vi "CH1603_OFF All Relay.vi"(5 "Loop Read(3)":i32=3, 7 "Device Addr(0x01)":u8=1 format="%02x", 8 "error in (no error)":errorcluster, 9 "Delay Time(200ms)":u32=200, 11 "MyIndex":u8) -> (0 "error out":errorcluster, 2 "Result(T:Pass)":bool, 3 "VISA resource name out":refnum<visa-resource-name>)   [LabVIEW 2015]
doc: "Close the device all IO port(1~16 or 17~32),will set the second device IO(device address add 1);"
panel:
  out "Read String":string
  # "OFF All IO Port"
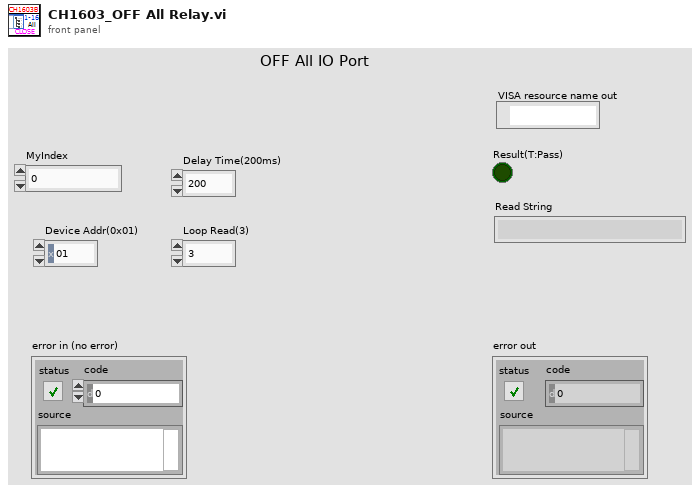
[diagram p1: front panel]
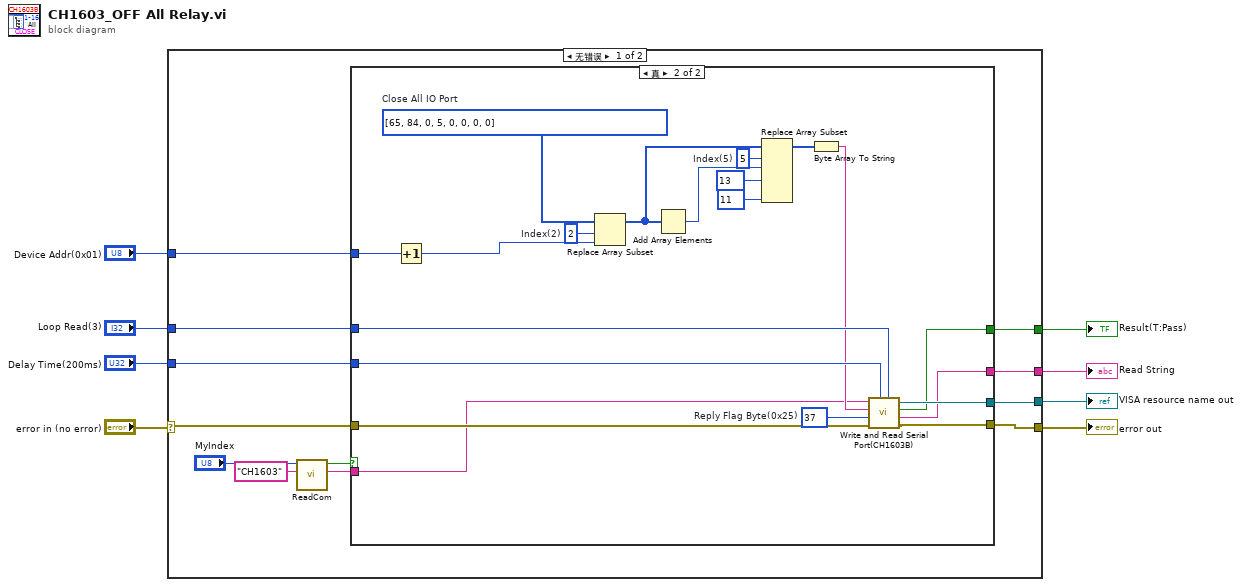
[diagram p0: block diagram]
diagram:
  n1 = case shown="无错误" "error in (no error)" {
    selector: "error in (no error)" -> [w19 w41]
    tunnel: [w18 w41] -> w6
    tunnel: [w17 _] -> w7
    tunnel: "Device Addr(0x01)" -> [w20 _]
    tunnel: "Delay Time(200ms)" -> [w16 _]
    tunnel: "Loop Read(3)" -> [w15 _]
    tunnel: [w14 _] -> w2
    tunnel: [w13 _] -> w1
    frame No Error {
      n2 = call "ReadCom.vi"("仪器名称"="CH1603", "MyIndex"="MyIndex") -> ("COM"=w9:string, "OK?"=w10:bool)  [unwired: 7 in, 1 out]
      n3 = case shown="真" w10 {
        tunnel: w20 -> [_ w34]
        tunnel: w19 -> [_ w33]
        tunnel: [_ w32] -> w18
        tunnel: [_ w31] -> w17
        tunnel: w16 -> [_ w30]
        tunnel: w15 -> [_ w29]
        tunnel: [_ w24] -> w14
        tunnel: [_ w23] -> w13
        tunnel: w9 -> [_ w21]
        frame False {
        }
        frame True {
          w25 = u8 37  # Reply Flag Byte(0x25)
          w38 = 5  # Index(5)
          w39 = 2  # Index(2)
          w40 = u8[] [65, 84, 0, 5, 0, 0, 0, 0]  # Close All IO Port
          n4 = Increment(x=w34) -> (x+1=w22:u8)
          n5 = Replace Array Subset(array=w40, new element=w22, index=w39) -> (w28:u8[])
          n6 = Add Array Elements(numeric array=w28) -> (sum=w27:u8)
          n7 = Replace Array Subset(array=w28, new element #1=w27, index #1=w38, new element #2=u8 13 ("Device Addr(0x01) 2"), new element #3=u8 11 ("Device Addr(0x01) 2")) -> (w35:u8[])  [unwired: 2 in]
          n8 = Byte Array To String(unsigned byte array=w35) -> (string=w26:string)
          n9 = call "Write and Read Serial Port(CH1603B).vi"("Loop Read(3)"=w29, "Delay Time(200ms)"=w30, "error in (no error)"=w33, "Reply Flag Byte"=w25, "Write Command"=w26, "VISA resource name in"=w21) -> ("error out"=w32:errorcluster, "Read String"=w23:string, "Result(T:Pass)"=w24:bool, "VISA resource name out"=w31:refnum<visa-resource-name>)  [unwired: 2 in]
        }
      }
    }
    frame Error {
    }
  }
  "VISA resource name out" <- w7
  "error out" <- w6
  "Result(T:Pass)" <- w2
  "Read String" <- w1
